vi "UHR-Fleezers Control (host) - 12.0_test_fpga_connection.vi"() -> ()   [LabVIEW 2014] (continued)
            n1532 = VISA Write(VISA resource name=w2158, write buffer=w2147) -> (VISA resource name out=w2146:refnum<visa-resource-name>)  [unwired: 1 in, 2 out]
            n1533 = Concatenate Strings("cvolume" ("string"), "\r") -> (w2145:string)
            n1534 = VISA Write(VISA resource name=w2146, write buffer=w2145) -> (VISA resource name out=w2156:refnum<visa-resource-name>)  [unwired: 1 in, 2 out]
            n1535 = Concatenate Strings("irun" ("string"), "\r") -> (w2154:string)
            n1536 = VISA Write(VISA resource name=w2156, write buffer=w2154) -> ()  [unwired: 1 in, 3 out]
          }
          frame #1 {
            "Flushing P3" <- TRUE ("Flushing P3")
          }
        }
      }
      event "Flush Pump 1": Value Change {
        n1537 = event-data() -> ()  [unwired: 7 out]
        n1538 = flat-sequence {
          tunnel: [w2176] -> w2166
          tunnel: w2165 -> [w2169]
          tunnel: w2166 -> [_]
          frame #0 {
            # "set paramaters (rate, volume) for flush, clear volume"
            n1539 = local write "Inject Pump 1"(TRUE ("Inject Pump 1")) -> ()
            n1540 = Number To Decimal String(number="Flush rate (uL/m) P1") -> (decimal integer string=w2192:string)  [unwired: 1 in]
            n1541 = Concatenate Strings("irate  " ("string"), w2192, " u/m" ("string"), "\r") -> (w2194:string)
            n1542 = VISA Write(VISA resource name=w2169, write buffer=w2194) -> (VISA resource name out=w2190:refnum<visa-resource-name>)  [unwired: 1 in, 2 out]
            n1543 = Reciprocal(x="Flush rate (uL/m) P1") -> (1/x=w2173:dbl)
            n1544 = Number To Decimal String(number="Volume (uL) P1") -> (decimal integer string=w2181:string)  [unwired: 1 in]
            n1545 = Multiply(x="Volume (uL) P1", y=w2173) -> (x*y=w2172:dbl)
            n1546 = Concatenate Strings("tvolume  " ("string"), w2181, " u" ("string"), "\r") -> (w2179:string)
            n1547 = Multiply(x=w2172, y=60.0) -> (x*y=→"HP1 Flush Time (s)":dbl)
            n1548 = VISA Write(VISA resource name=w2190, write buffer=w2179) -> (VISA resource name out=w2178:refnum<visa-resource-name>)  [unwired: 1 in, 2 out]
            n1549 = Concatenate Strings("cvolume" ("string"), "\r") -> (w2177:string)
            n1550 = VISA Write(VISA resource name=w2178, write buffer=w2177) -> (VISA resource name out=w2188:refnum<visa-resource-name>)  [unwired: 1 in, 2 out]
            n1551 = Concatenate Strings("irun" ("string"), "\r") -> (w2186:string)
            n1552 = VISA Write(VISA resource name=w2188, write buffer=w2186) -> (VISA resource name out=w2176:refnum<visa-resource-name>)  [unwired: 1 in, 2 out]
          }
          frame #1 {
            "Flushing P1" <- TRUE ("Flushing P3")
          }
        }
      }
      event "Clear Volume": Value Change {
        n1553 = event-data() -> ()  [unwired: 7 out]
        n1554 = Number To Decimal String(number="Normal volume (mL)") -> (decimal integer string=w2201:string)  [unwired: 1 in]
        n1555 = Concatenate Strings("tvolume " ("string"), w2201, " u" ("string"), "\r") -> (w2198:string)
        n1556 = VISA Write(VISA resource name=w2204, write buffer=w2198) -> (VISA resource name out=w2197:refnum<visa-resource-name>)  [unwired: 1 in, 2 out]
        n1557 = local write "Clear Volume"(FALSE ("Clear Volume")) -> ()
        n1558 = Concatenate Strings("cvolume" ("string"), "\r") -> (w2206:string)
        n1559 = VISA Write(VISA resource name=w2197, write buffer=w2206) -> ()  [unwired: 1 in, 3 out]
      }
      event "Clear Volume P3": Value Change {
        n1560 = event-data() -> ()  [unwired: 7 out]
        n1561 = Concatenate Strings("cvolume" ("string"), "\r") -> (w2212:string)
        n1562 = VISA Write(VISA resource name=w2211, write buffer=w2212) -> ()  [unwired: 1 in, 3 out]
        n1563 = local write "Clear Volume P3"(FALSE ("Clear Volume P3")) -> ()
      }
      event "Clear Volume P1": Value Change {
        n1564 = event-data() -> ()  [unwired: 7 out]
        n1565 = Concatenate Strings("cvolume" ("string"), "\r") -> (w2217:string)
        n1566 = local write "Clear Volume P1"(FALSE ("Clear Volume P1")) -> ()
        n1567 = VISA Write(VISA resource name=w2216, write buffer=w2217) -> ()  [unwired: 1 in, 3 out]
      }
      event "Display On P3": Value Change {
        n1568 = event-data() -> ()  [unwired: 7 out]
        n1569 = Select(t="dim 100", s="Display On P3", f="dim 0") -> (s? t:f=w2223:string)
        n1570 = Concatenate Strings(w2223, "\r") -> (w2225:string)
        n1571 = VISA Write(VISA resource name=w2220, write buffer=w2225) -> ()  [unwired: 1 in, 3 out]
      }
      event "Display On P1": Value Change {
        n1572 = event-data() -> ()  [unwired: 7 out]
        n1573 = Select(t="dim 100", s="Display On P1", f="dim 0") -> (s? t:f=w2230:string)
        n1574 = Concatenate Strings(w2230, "\r") -> (w2232:string)
        n1575 = VISA Write(VISA resource name=w2227, write buffer=w2232) -> ()  [unwired: 1 in, 3 out]
      }
      event "Retract Pump 3": Value Change {
        n1576 = event-data() -> ()  [unwired: 7 out]
        n1577 = local write "Retract Pump 3"(FALSE ("Retract Pump 3")) -> ()
        n1578 = case shown="True" "Retract Pump 3" {
          tunnel: w2234 -> [_ w2237]
          frame False {
          }
          frame True {
            n1579 = Number To Decimal String(number="Retract Rate (mL/m)") -> (decimal integer string=w2255:string)  [unwired: 1 in]
            n1580 = Concatenate Strings("wrate  " ("string"), w2255, " u/m" ("string"), "\r") -> (w2257:string)
            n1581 = VISA Write(VISA resource name=w2237, write buffer=w2257) -> (VISA resource name out=w2248:refnum<visa-resource-name>)  [unwired: 1 in, 2 out]
            n1582 = Number To Decimal String(number="Retract Vol 3 (uL)") -> (decimal integer string=w2250:string)  [unwired: 1 in]
            n1583 = Concatenate Strings("tvolume  " ("string"), w2250, " u" ("string"), "\r") -> (w2247:string)
            n1584 = VISA Write(VISA resource name=w2248, write buffer=w2247) -> (VISA resource name out=w2243:refnum<visa-resource-name>)  [unwired: 1 in, 2 out]
            n1585 = Concatenate Strings("cvolume" ("string"), "\r") -> (w2244:string)
            n1586 = VISA Write(VISA resource name=w2243, write buffer=w2244) -> (VISA resource name out=w2238:refnum<visa-resource-name>)  [unwired: 1 in, 2 out]
            n1587 = Concatenate Strings("wrun" ("string"), "\r") -> (w2239:string)
            n1588 = VISA Write(VISA resource name=w2238, write buffer=w2239) -> ()  [unwired: 1 in, 3 out]
          }
        }
      }
      event "Retract Pump 1": Value Change {
        n1589 = event-data() -> ()  [unwired: 7 out]
        n1590 = local write "Retract Pump 1"(FALSE ("Retract Pump 1")) -> ()
        n1591 = case shown="True" "Retract Pump 1" {
          tunnel: w2259 -> [_ w2264]
          frame False {
          }
          frame True {
            n1592 = local read "Retract Rate (mL/m)"() -> (w2262:dbl)
            n1593 = Number To Decimal String(number=w2262) -> (decimal integer string=w2280:string)  [unwired: 1 in]
            n1594 = Concatenate Strings("wrate  " ("string"), w2280, " u/m" ("string"), "\r") -> (w2282:string)
            n1595 = VISA Write(VISA resource name=w2264, write buffer=w2282) -> (VISA resource name out=w2274:refnum<visa-resource-name>)  [unwired: 1 in, 2 out]
            n1596 = Number To Decimal String(number="Retract Vol 1 (uL)") -> (decimal integer string=w2276:string)  [unwired: 1 in]
            n1597 = Concatenate Strings("tvolume  " ("string"), w2276, " u" ("string"), "\r") -> (w2273:string)
            n1598 = VISA Write(VISA resource name=w2274, write buffer=w2273) -> (VISA resource name out=w2270:refnum<visa-resource-name>)  [unwired: 1 in, 2 out]
            n1599 = Concatenate Strings("cvolume" ("string"), "\r") -> (w2271:string)
            n1600 = VISA Write(VISA resource name=w2270, write buffer=w2271) -> (VISA resource name out=w2265:refnum<visa-resource-name>)  [unwired: 1 in, 2 out]
            n1601 = Concatenate Strings("wrun" ("string"), "\r") -> (w2266:string)
            n1602 = VISA Write(VISA resource name=w2265, write buffer=w2266) -> ()  [unwired: 1 in, 3 out]
          }
        }
      }
      event "Flip Green Filter": Value Change {
        n1603 = event-data() -> ()  [unwired: 7 out]
        n1604 = Not(x="Flip Green Filter") -> (.not. x?=w2284:bool)
        n1605 = local write "Flip Green Filter"(w2284) -> ()
        n1606 = flat-sequence {
          tunnel: w2292 -> [w2297]
          tunnel: w2291 -> [w2296]
          tunnel: [w2294] -> w2289
          tunnel: [w2293] -> w2288
          tunnel: [w2299] -> w2287
          tunnel: w2289 -> [w2299]
          tunnel: [w2298] -> w2286
          tunnel: w2288 -> [w2298]
          tunnel: w2287 -> [w2303]
          tunnel: w2286 -> [w2302]
          tunnel: [w2301] -> w2290
          frame #0 {
            n1607 = xnode "Read/Write Control"("FPGA VI Reference In"=w2297, "error in"=w2296, "Green Filter Flipper"=TRUE) -> ("FPGA VI Reference Out"=w2294:T22, "error out"=w2293:errorcluster)
          }
          frame #1 {
            n1608 = Wait (ms)(milliseconds to wait=u32 100) -> ()  [unwired: 1 out]
          }
          frame #2 {
            n1609 = xnode "Read/Write Control"("FPGA VI Reference In"=w2303, "error in"=w2302, "Green Filter Flipper"=FALSE) -> ("error out"=w2301:errorcluster)  [unwired: 1 out]
          }
        }
      }
      event "Pump 1 contents", "Pump 3 contents": Value Change {
        n1610 = event-data() -> ()  [unwired: 7 out]
        n1611 = local read "Pump 1 contents"() -> (→"Pump 1 cont disp":string)
        n1612 = local read "Pump 3 contents"() -> (→"Pump 3 cont disp":string)
      }
      event "Reset Trap Pos. FB": Value Change {
        n1613 = event-data() -> ()  [unwired: 7 out]
        n1614 = xnode "Read/Write Control"("FPGA VI Reference In"=w2309, "error in"=w2308, "Trap Pos. FB Reset"="Reset Trap Pos. FB") -> ()  [unwired: 2 out]
      }
      event "Rem fb disp offset": Value Change {
        n1615 = event-data() -> ()  [unwired: 7 out]
        n1616 = local write "Rem fb disp offset"(FALSE ("Rem fb disp offset")) -> ()
        n1617 = local read "Mean T1 Position (nm)"() -> (w2311:dbl)
        n1618 = local read "FB Trap Pos Offset"() -> (w2312:dbl)
        n1619 = Subtract(x=w2312, y=w2311) -> (x-y=w2310:dbl)
        n1620 = local write "FB Trap Pos Offset"(w2310) -> ()
      }
      event "Threshold (nm)": Value Change {
        n1621 = event-data() -> ()  [unwired: 7 out]
        n1622 = flat-sequence {
          tunnel: w2316 -> [w2324]
          tunnel: w2315 -> [w2323]
          tunnel: [w2317] -> w2314
          tunnel: w2314 -> [w2330]
          frame #0 {
            n1623 = xnode "Read/Write Control"("FPGA VI Reference In"=w2324, "error in"=w2323) -> ("FPGA VI Reference Out"=w2320:T22, "error out"=w2319:errorcluster, "FPGA TTrig Thresh"=w2321:i64)
            n1624 = local read "Threshold stored (nm)"() -> (w2329:dbl)
            n1625 = local read "Threshold (nm)"() -> (w2317:dbl)
            n1626 = local read "AOM X Cal (nm/MHz)"() -> (w2327:dbl)
            n1627 = Subtract(x=w2317, y=w2329) -> (x-y=w2328:dbl)
            n1628 = Divide(x=w2328, y=w2327) -> (x/y=w2325:dbl)
            n1629 = call "IR AOM freq to word.vi"("Frequency In (MHz)"=w2325) -> ("Frequency Word Out (double)"=w2326:dbl)
            n1630 = To Quad Integer(1:w2326) -> (0:w2322:i64)
            n1631 = Add(x=w2321, y=w2322) -> (x+y=w2318:i64)
            n1632 = xnode "Read/Write Control"("FPGA VI Reference In"=w2320, "error in"=w2319, "FPGA TTrig Thresh"=w2318) -> ()  [unwired: 2 out]
          }
          frame #1 {
            "Threshold stored (nm)" <- w2330
          }
        }
      }
      event "FB Trig Integrate": Value Change {
        n1633 = event-data() -> ()  [unwired: 7 out]
        n1634 = local read "FB Trig Integrate"() -> (w2332:u32)
        n1635 = xnode "Read/Write Control"("FPGA VI Reference In"=w2334, "error in"=w2333, "FB Trig Integrate"=w2332) -> ("error out"=w2331:errorcluster)  [unwired: 1 out]
      }
      event "11": Value Change {
        n1636 = event-data() -> ()  [unwired: 7 out]
        n1637 = local read "11"() -> (w2335:bool)
        n1638 = case shown="True" w2335 {
          frame False {
          }
          frame True {
            n1639 = local read "Messages"() -> (w2337:string)
            n1640 = call "Update messages.vi"("Message to add"="You kicked it up to 11!", "Old message string"=w2337) -> ("New message string"=w2338:string)
            n1641 = call <vilib>:"Beep.vi"() -> ()  [unwired: 12 in]
            n1642 = local write "Messages"(w2338) -> ()
          }
        }
      }
      event "Trap Pos. FB ON": Value Change {
        n1643 = event-data() -> ()  [unwired: 7 out]
        n1644 = xnode "Read/Write Control"("FPGA VI Reference In"=w2341, "error in"=w2340, "Force feedback"="Trap Pos. FB ON") -> ()  [unwired: 2 out]
      }
      event "Remove Action Offset": Value Change {
        n1645 = event-data() -> ()  [unwired: 7 out]
        n1646 = local write "Remove Action Offset"(FALSE ("Remove Action Offset")) -> ()
        n1647 = local read "Trap Pos. FB Mult Factor"() -> (w2346:i64)
        n1648 = local read "Trap Pos FB Action"() -> (w2344:i64)
        n1649 = local read "Trap Pos. FB Offset Factor"() -> (w2342:i64)
        n1650 = Multiply(x=w2346, y=w2344) -> (x*y=w2345:i64)
        n1651 = Add(x=w2345, y=w2342) -> (x+y=w2343:i64)
        n1652 = local write "Trap Pos. FB Offset Factor"(w2343) -> ()
        n1653 = xnode "Read/Write Control"("FPGA VI Reference In"=w2349, "error in"=w2348, "Trap Pos. FB Offset Factor"=w2343) -> ()  [unwired: 2 out]
      }
      event "Remove Offset to factor": Value Change {
        n1654 = event-data() -> ()  [unwired: 7 out]
        n1655 = local write "Remove Offset to factor"(FALSE ("Remove Action Offset")) -> ()
        n1656 = local read "Trap Pos. FB Mult Factor"() -> (w2361:i64)
        n1657 = local read "Trap Pos FB Action"() -> (w2359:i64)
        n1658 = local read "Trap Pos. FB Offset Factor"() -> (w2358:i64)
        n1659 = Multiply(x=w2361, y=w2359) -> (x*y=w2360:i64)
        n1660 = local read "Trap Pos. FB Mult Factor"() -> (w2357:i64)
        n1661 = Add(x=w2360, y=w2358) -> (x+y=w2352:i64)
        n1662 = Multiply(x=32768, y="factor") -> (x*y=w2355:dbl)
        n1663 = Multiply(x=w2355, y=w2357) -> (x*y=w2356:dbl)
        n1664 = Subtract(x=w2352, y=w2356) -> (x-y=w2350:dbl)
        n1665 = To Quad Integer(1:w2350) -> (0:w2351:i64)
        n1666 = xnode "Read/Write Control"("FPGA VI Reference In"=w2364, "error in"=w2363, "Trap Pos. FB Offset Factor"=w2351) -> ()  [unwired: 2 out]
        n1667 = local write "Trap Pos. FB Offset Factor"(w2351) -> ()
      }
      event "Trap Pos. FB Range", "Trap Pos. FB Gains", "Trap Pos. FB Mult Factor", "Trap Pos. FB Offset Factor", "Trap Pos FB Negate Action", "Trap Pos FB Monitor\nT1 or T2", "Differential FB?", "Negate Diff?": Value Change {
        n1668 = event-data() -> ()  [unwired: 7 out]
        n1669 = local read "Negate Diff?"() -> (w2365:bool)
        n1670 = xnode "Read/Write Control"("FPGA VI Reference In"=w2375, "error in"=w2374, "Trap Pos. FB Range"="Trap Pos. FB Range", "Trap Pos. FB Gains"="Trap Pos. FB Gains", "Trap Pos. FB Mult Factor"="Trap Pos. FB Mult Factor", "Trap Pos. FB Offset Factor"="Trap Pos. FB Offset Factor", "Trap Pos FB Negate Action"="Trap Pos FB Negate Action", "Trap Pos FB Monitor T1 or T2"="Trap Pos FB Monitor\nT1 or T2", "AI1 X Scale"="Trap Pos. AI1 X Pre-scale", "Negate Diff?"=w2365, "Diff FB Measurement?"="Differential FB?") -> ()  [unwired: 2 out]
      }
      event "Trap Pos FB SP", "Trap Pos FB SP 2", "Use SP 2": Value Change {
        n1671 = event-data() -> ()  [unwired: 7 out]
        n1672 = Select(t="Trap Pos FB SP 2", s="Use SP 2", f="Trap Pos FB SP") -> (s? t:f=w2376:fxp<+/-,16,1>)
        n1673 = xnode "Read/Write Control"("FPGA VI Reference In"=w2381, "error in"=w2380, "Trap Pos. FB SP"=w2376) -> ()  [unwired: 2 out]
      }
      event "Offset SP2 from SP1": Value Change {
        n1674 = event-data() -> ()  [unwired: 7 out]
        n1675 = local read "Trap Pos FB SP"() -> (w2384:fxp<+/-,16,1>)
        n1676 = Add(x=w2384, y="SP2 Offset") -> (x+y=w2382:fxp<+/-,16,1>)
        n1677 = property on="Trap Pos FB SP 2" class="DigNum (strict)"("Val(Sgnl)"=w2382) -> ()  [unwired: 2 in, 2 out]
        n1678 = local write "Offset SP2 from SP1"(FALSE ("Offset SP2 from SP1")) -> ()
      }
      event "Set Reading to\nSetpoint": Value Change {
        # "This is the actual PID input signal"
        n1679 = event-data() -> ()  [unwired: 7 out]
        n1680 = local write "Set Reading to\nSetpoint"(FALSE ("Set SP to Reading")) -> ()
        n1681 = xnode "Read/Write Control"("FPGA VI Reference In"=w2390, "error in"=w2389) -> ("FPGA VI Reference Out"=w2388:T22, "error out"=w2387:errorcluster, "Trap Pos FB Int-Norm Signal"=w2386:fxp<+/-,16,1>)
        n1682 = local read "Differential FB?"() -> (w2391:bool)
        n1683 = case shown="False" w2391 {
          tunnel: [w2396 w2403] -> w2393
          tunnel: w2386 -> [w2394 w2403]
          frame False {
            n1684 = local read "Trap Pos FB Monitor\nT1 or T2"() -> (w2399:bool)
            n1685 = local read "Trap X AI1 (DMA)"() -> (w2402:T13)
            n1686 = Unbundle By Name(w2402) -> ("Set 1"=w2401:fxp<+/-,16,1>, "Set 2"=w2400:fxp<+/-,16,1>)
            n1687 = Select(t=w2401, s=w2399, f=w2400) -> (s? t:f=w2398:fxp<+/-,16,1>)
            n1688 = Not(x="Set SP Using...") -> (.not. x?=w2395:bool)
            n1689 = Select(t=w2394, s=w2395, f=w2398) -> (s? t:f=w2396:fxp<+/-,16,1>)
          }
          frame True {
          }
        }
        n1690 = xnode "Read/Write Control"("FPGA VI Reference In"=w2388, "error in"=w2387, "Trap Pos. FB SP"=w2393) -> ()  [unwired: 2 out]
        n1691 = local write "Trap Pos FB SP"(w2393) -> ()
      }
      event "Trap Pos. FB Out Scale 2^n": Value Change {
        n1692 = event-data() -> ()  [unwired: 7 out]
        n1693 = Scale By Power Of 2(n="Trap Pos. FB Out Scale 2^n", x=ext 1.0) -> (x*2^n=w2404:ext)
        n1694 = property on="Trap Pos. FB Mult Factor" class="DigNum (strict)"("Val(Sgnl)"=w2404) -> ()  [unwired: 2 in, 2 out]
      }
      event "Trap Pos FB Int Count": Value Change {
        n1695 = event-data() -> ()  [unwired: 7 out]
        n1696 = xnode "Read/Write Control"("FPGA VI Reference In"=w2409, "error in"=w2408, "Trap Pos FB Int Count"="Trap Pos FB Int Count") -> ()  [unwired: 2 out]
      }
      event "Trap pos": Value Change {
        n1697 = event-data() -> ()  [unwired: 7 out]
        n1698 = case shown="True" "Trap pos" {
          frame False {
            n1699 = property on="Trap Delta Graph" class="WFGraph (strict)"("Visible"=TRUE) -> ()  [unwired: 2 in, 2 out]
            n1700 = property on="Saved trap pos" class="WFGraph (strict)"("Visible"=FALSE) -> ()  [unwired: 2 in, 2 out]
          }
          frame True {
            n1701 = property on="Saved trap pos" class="WFGraph (strict)"("Visible"=TRUE) -> ()  [unwired: 2 in, 2 out]
            n1702 = property on="Trap Delta Graph" class="WFGraph (strict)"("Visible"=FALSE) -> ()  [unwired: 2 in, 2 out]
          }
        }
      }
      event "Save user params": Value Change {
        n1703 = event-data() -> ()  [unwired: 7 out]
        n1704 = local write "Save user params"(FALSE ("Save user\nparams")) -> ()
        n1705 = call "save control values.vi"("User"="User") -> ()  [unwired: 8 in, 1 out]
        n1706 = local read "Messages"() -> (w2421:string)
        n1707 = Concatenate Strings("User: ", "User", "\r", "Parameters saved.") -> (w2416:string)
        n1708 = call "Update messages.vi"("Message to add"=w2416, "Old message string"=w2421) -> ("New message string"=w2415:string)
        n1709 = local write "Messages"(w2415) -> ()
      }
      event "Load user params": Value Change {
        n1710 = event-data() -> ()  [unwired: 7 out]
        n1711 = local write "Load user params"(FALSE ("Read user\nparams")) -> ()
        n1712 = flat-sequence {
          tunnel: [w2453] -> w2441
          tunnel: [w2452] -> w2439
          tunnel: [w2451] -> w2437
          tunnel: [w2450] -> w2435
          tunnel: [w2449] -> w2433
          tunnel: [w2448] -> w2431
          tunnel: [w2447] -> w2429
          tunnel: [w2446] -> w2427
          tunnel: [w2445] -> w2425
          tunnel: [w2444] -> w2423
          tunnel: [w2463] -> w2442
          tunnel: w2441 -> [w2463]
          tunnel: [w2462] -> w2440
          tunnel: w2439 -> [w2462]
          tunnel: [w2461] -> w2438
          tunnel: w2437 -> [w2461]
          tunnel: [w2460] -> w2436
          tunnel: w2435 -> [w2460]
          tunnel: [w2459] -> w2434
          tunnel: w2433 -> [w2459]
          tunnel: [w2458] -> w2432
          tunnel: w2431 -> [w2458]
          tunnel: [w2457] -> w2430
          tunnel: w2429 -> [w2457]
          tunnel: [w2456] -> w2428
          tunnel: w2427 -> [w2456]
          tunnel: [w2455] -> w2426
          tunnel: w2425 -> [w2455]
          tunnel: [w2454] -> w2424
          tunnel: w2423 -> [w2454]
          tunnel: w2442 -> [w2480]
          tunnel: w2440 -> [w2479]
          tunnel: w2438 -> [w2478]
          tunnel: w2436 -> [w2477]
          tunnel: w2434 -> [w2476]
          tunnel: w2432 -> [w2475]
          tunnel: w2430 -> [w2474]
          tunnel: w2428 -> [w2473]
          tunnel: w2426 -> [w2472]
          tunnel: w2424 -> [w2471]
          frame #0 {
            # "Make exceptions.\nThese will not be\nloaded."
            n1713 = local read "Sample Channel\nFlow"() -> (w2448:bool)
            n1714 = local read "Green ON/Interlacing"() -> (w2449:bool)
            n1715 = local read "Trap 1 (ON/OFF)"() -> (w2453:bool)
            n1716 = local read "Trap 2 (ON/OFF)"() -> (w2452:bool)
            n1717 = local read "Trap Pos. FB ON"() -> (w2444:bool)
            n1718 = local read "Inject Pump 1"() -> (w2447:bool)
            n1719 = local read "Inject Pump 3"() -> (w2446:bool)
            n1720 = local read "Trap D (MHz)"() -> (w2445:dbl)
            n1721 = local read "Index"() -> (w2450:dbl)
            n1722 = local read "Fish"() -> (w2451:bool)
          }
          frame #1 {
            n1723 = local read "User"() -> (w2464:string)
            n1724 = call "retrieve control values.vi"("User"=w2464) -> ()  [unwired: 10 in, 1 out]
            n1725 = local read "Messages"() -> (w2470:string)
            n1726 = Concatenate Strings("User: ", w2464, "\r", "Parameters loaded.") -> (w2465:string)
            n1727 = call "Update messages.vi"("Message to add"=w2465, "Old message string"=w2470) -> ("New message string"=w2469:string)
            n1728 = local write "Messages"(w2469) -> ()
          }
          frame #2 {
            n1729 = local write "Sample Channel\nFlow"(w2475) -> ()
            n1730 = local write "Green ON/Interlacing"(w2476) -> ()
            n1731 = local write "Trap 1 (ON/OFF)"(w2480) -> ()
            n1732 = local write "Trap 2 (ON/OFF)"(w2479) -> ()
            n1733 = local write "Inject Pump 1"(w2474) -> ()
            n1734 = local write "Trap Pos. FB ON"(w2471) -> ()
            n1735 = local write "Inject Pump 3"(w2473) -> ()
            n1736 = local write "Trap D (MHz)"(w2472) -> ()
            n1737 = local write "Index"(w2477) -> ()
            n1738 = local write "Fish"(w2478) -> ()
          }
        }
      }
      event "Abort wiggle": Value Change {
        n1739 = event-data() -> ()  [unwired: 7 out]
        n1740 = flat-sequence {
          tunnel: w2484 -> [w2488]
          tunnel: w2483 -> [w2487]
          tunnel: [w2486] -> w2481
          tunnel: [w2490] -> w2482
          tunnel: w2481 -> [w2490]
          frame #0 {
            n1741 = xnode "Read/Write Control"("FPGA VI Reference In"=w2488, "error in"=w2487, "Abort wiggle 1"="Abort wiggle", "Abort wiggle 2"="Abort wiggle") -> ("error out"=w2486:errorcluster)  [unwired: 1 out]
          }
          frame #1 {
            n1742 = local write "Abort wiggle"(FALSE ("Abort wiggle")) -> ()
          }
        }
      }
    }
    "error out 2" <- w1261
    n1743 = node-c288() -> ()  [unwired: 2 out]
  }
  n1744 = node-c288() -> (w126:T26)  [unwired: 4 in]
  n1745 = local write "Target size"(cluster{"Width":dbl, "Height":dbl} {"Width"=40.0, "Height"=40.0} ("Target size")) -> ()
  n1746 = timed-loop "Run Scripts, including: stage motion" {
    tunnel: w130 -> [w2498]
    tunnel: w5 -> [w2499]
    tunnel: [w2499] -> w129
    tunnel: [w2498] -> w128
    timing: w126 -> [_]
    timing-out: [_] -> w125
    tunnel: w111 -> [w2497]
    tunnel: w112 -> [w2496]
    tunnel: w55 -> [w2493]
    tunnel: w54 -> [w2492]
    tunnel: w53 -> [w2494]
    tunnel: w52 -> [w2495]
    stop <- w2491 stop-if-true
    n1747 = node-c288() -> ()  [unwired: 1 in, 1 out]
    n1748 = event shown="[12] \"Got ADig bead\": Value Change" {
      selector: _ -> [_ _ _ _ _ _ _ _ _ _ _ _ _ _ _ _ _ _ _ _ _]
      dyn-events: _ -> [_ _ _ _ _ _ _ _ _ _ _ _ _ _ _ _ _ _ _ _ _]
      timeout: _ -> [_ _ _ _ _ _ _ _ _ _ _ _ _ _ _ _ _ _ _ _ _]
      tunnel: ["Set Position" "Move to Position" _ _ "Read Harvard" _ _ _ _ _ _ _ "Got ADig bead" "Force FB Script" "Rupture Script" _ "Got DNA bead" "Take Stepping Data" _ "Take Detection Laser\nImage" _] -> _
      tunnel: [_ _ _ _ _ _ _ _ _ _ _ _ _ _ _ _ _ _ _ _ w3172] -> w2491
      tunnel: w2498 -> [w2517 w2525 w2538 w2568 _ w2616 w2656 w2739 w2770 w2904 w2930 w2965 _ w2983 _ _ _ _ _ _ _]
      tunnel: w2499 -> [w2518 w2526 w2539 w2569 _ w2617 w2657 w2740 w2771 w2905 w2931 w2966 _ w2984 _ _ _ _ _ _ _]
      tunnel: w2497 -> [_ _ _ _ w2601 _ _ _ _ _ _ _ _ _ _ _ _ _ _ _ _]
      tunnel: w2496 -> [_ _ _ _ w2600 _ _ _ _ _ _ _ _ _ _ _ _ _ _ _ _]
      tunnel: w2495 -> [_ _ _ _ _ _ _ _ _ _ _ _ _ _ _ _ _ _ _ _ _]
      tunnel: w2494 -> [_ _ _ _ _ _ _ _ _ _ _ _ _ _ _ _ _ _ _ _ _]
      tunnel: w2493 -> [_ _ _ _ _ _ _ _ _ _ _ _ _ _ _ _ _ _ _ _ _]
      tunnel: w2492 -> [_ _ _ _ _ _ _ _ _ _ _ _ _ _ _ _ _ _ _ _ _]
      event "Set Position", "Set Position 2", "Set Position 3", "Set Position 4", "Set Position 5", "Set Position 1": Value Change {
        n1749 = event-data() -> ()  [unwired: 1 in, 5 out]
        n1750 = Build Array("Set Position 1", "Set Position 2", "Set Position 3", "Set Position 4", "Set Position 5") -> (w2516:bool[])
        n1751 = Boolean Array To Number(Boolean array=w2516) -> (number=w2515:u32)
        n1752 = Logarithm Base 2(1:w2515) -> (0:w2507:dbl)
        n1753 = call "Read Stage Position.vi"("error in"=w2517, "VISA resource name in"=w2518) -> ("Current Position"=w2522:cluster{dbl, dbl, dbl}, "error out"=w2521:errorcluster)  [unwired: 2 out]
        n1754 = Decrement(x="Position") -> (x-1=w2505:dbl)
        n1755 = Greater Or Equal?(x=w2507, y=0.0) -> (x >= y?=w2508:bool)
        n1756 = Cluster To Array(cluster=w2522) -> (array=w2519:dbl[])
        n1757 = local write "Stage Control Serial Error"(w2521) -> ()
        n1758 = Select(t=w2507, s=w2508, f=w2505) -> (s? t:f=w2504:dbl)
        n1759 = Increment(x=w2504) -> (x+1=w2503:dbl)
        n1760 = Build Array (concatenate)(w2503, w2519) -> (w2502:dbl[])
        n1761 = Replace Array Subset(array="Saved Stage Positions", new element=w2502, index (row)=w2504) -> (w2520:dbl[][])  [unwired: 1 in]
        n1762 = local write "Saved Stage Positions"(w2520) -> ()
      }
      event "Move to Position": Value Change {
        n1763 = event-data() -> ()  [unwired: 1 in, 5 out]
        n1764 = flat-sequence {
          tunnel: w2526 -> [w2530]
          tunnel: w2525 -> [w2529]
          frame #0 {
            n1765 = local read "Saved Stage Positions"() -> (w2532:dbl[][])
            n1766 = local read "Position"() -> (w2531:dbl)
            n1767 = local write "Stage Moving"(TRUE ("Stage Moving")) -> ()
            n1768 = call "move to saved stage position.vi"("error in"=w2529, "Stage VISA resource name in"=w2530, "Position"=w2531, "Saved Stage Positions"=w2532) -> ("error out"=w2528:errorcluster)  [unwired: 1 out]
            n1769 = local write "Stage Control Serial Error"(w2528) -> ()
          }
          frame #1 {
            n1770 = call <vilib>:"Beep.vi"() -> ()  [unwired: 3 in, 9 out]
            n1771 = local write "Stage Moving"(FALSE ("Stage Moving")) -> ()
          }
        }
      }
      event "Move Cap. 1 (DNA Bottom)": Value Change {
        n1772 = event-data() -> ()  [unwired: 1 in, 5 out]
        n1773 = local write "Move Cap. 1 (DNA Bottom)"(FALSE ("Move Cap. 1 (DNA Right)")) -> ()
        n1774 = flat-sequence {
          tunnel: w2538 -> [w2541]
          tunnel: w2539 -> [w2542]
          tunnel: [w2542] -> w2536
          tunnel: [w2541] -> w2535
          tunnel: w2536 -> [w2544]
          tunnel: w2535 -> [w2543]
          frame #0 {
            n1775 = property on="Sample Channel\nFlow" class="Bool (strict)"("Val(Sgnl)"="Cap 1 Samp Flow ON") -> ()  [unwired: 2 in, 2 out]
          }
          frame #1 {
            n1776 = local read "Saved Stage Positions"() -> (w2554:dbl[][])
            n1777 = local write "Stage Moving"(TRUE ("Stage Moving")) -> ()
            n1778 = Array Subset(array=w2554, index (row)=0 ("index"), length (row)=1 ("length"), index (col)=1 ("index"), length (col)=3 ("length")) -> (w2551:dbl[][])
            n1779 = Reshape Array(w2551, 3 ("dimension size")) -> (w2549:dbl[])
            n1780 = Array To Cluster(array=w2549) -> (cluster=w2548:cluster{"[0]":dbl, "[1]":dbl, "[2]":dbl})
            n1781 = call "Set Stage Position.vi"("Position"=w2548, "error in"=w2543, "VISA resource name in"=w2544) -> ("error out"=w2547:errorcluster)  [unwired: 2 out]
            n1782 = local write "Stage Control Serial Error"(w2547) -> ()
          }
          frame #2 {
            n1783 = local write "Stage Moving"(FALSE ("Stage Moving")) -> ()
            n1784 = case shown="True" "Cap 1 Flow ON" {
              frame False {
              }
              frame True {
                n1785 = property on="Inject Pump 1" class="Bool (strict)"("Val(Sgnl)"=TRUE ("Value (Signaling)")) -> ()  [unwired: 2 in, 2 out]
              }
            }
            n1786 = call <vilib>:"Beep.vi"() -> ()  [unwired: 3 in, 9 out]
          }
          frame #3 {
            n1787 = property on="Sample Channel\nFlow" class="Bool (strict)"("Val(Sgnl)"=FALSE ("Value (Signaling)")) -> ()  [unwired: 2 in, 2 out]
            n1788 = local read "Cap. 2 BD T1?\n(ADig T1, DNA T2)"() -> (w2561:bool)
            n1789 = case shown="True" w2561 {
              tunnel: "Cap 1 T ON" -> [w2563 w2564]
              frame False {
                n1790 = property on="Trap 1 (ON/OFF)" class="Bool (strict)"("Val(Sgnl)"=w2563) -> ()  [unwired: 2 in, 2 out]
              }
              frame True {
                n1791 = property on="Trap 2 (ON/OFF)" class="Bool (strict)"("Val(Sgnl)"=w2564) -> ()  [unwired: 2 in, 2 out]
              }
            }
            n1792 = property on="Got DNA bead" class="Bool (strict)"("Key Focus"=TRUE) -> ()  [unwired: 2 in, 2 out]
          }
        }
      }
      event "Move Cap. 2 (ADig Top)": Value Change {
        n1793 = event-data() -> ()  [unwired: 1 in, 5 out]
        n1794 = local write "Move Cap. 2 (ADig Top)"(FALSE ("Move Cap. 2 (ADig Left)")) -> ()
        n1795 = flat-sequence {
          tunnel: w2568 -> [w2571]
          tunnel: w2569 -> [w2572]
          tunnel: [w2572] -> w2566
          tunnel: [w2571] -> w2565
          tunnel: w2566 -> [w2574]
          tunnel: w2565 -> [w2573]
          frame #0 {
            n1796 = property on="Sample Channel\nFlow" class="Bool (strict)"("Val(Sgnl)"="Cap 2 Samp Flow ON") -> ()  [unwired: 2 in, 2 out]
          }
          frame #1 {
            n1797 = local read "Saved Stage Positions"() -> (w2584:dbl[][])
            n1798 = local write "Stage Moving"(TRUE ("Stage Moving")) -> ()
            n1799 = Array Subset(array=w2584, index (row)=1 ("index"), length (row)=1 ("length"), index (col)=1 ("index"), length (col)=3 ("length")) -> (w2581:dbl[][])
            n1800 = disable-structure shown="Disabled" {
              frame Disabled {
                w2586 = FALSE ("Value (Signaling)")
                n1801 = property on="Trap 1 (ON/OFF)" class="Bool (strict)"("Val(Sgnl)"=w2586) -> ()  [unwired: 2 in, 2 out]
                n1802 = property on="Trap 1 (ON/OFF)" class="Bool (strict)"("Val(Sgnl)"=w2586) -> ()  [unwired: 2 in, 2 out]
              }
              frame Enabled {
              }
            }
            n1803 = Reshape Array(w2581, 3 ("dimension size")) -> (w2579:dbl[])
            n1804 = Array To Cluster(array=w2579) -> (cluster=w2578:cluster{"[0]":dbl, "[1]":dbl, "[2]":dbl})
            n1805 = call "Set Stage Position.vi"("Position"=w2578, "error in"=w2573, "VISA resource name in"=w2574) -> ("error out"=w2577:errorcluster)  [unwired: 2 out]
            n1806 = local write "Stage Control Serial Error"(w2577) -> ()
          }
          frame #2 {
            n1807 = local write "Stage Moving"(FALSE ("Stage Moving")) -> ()
            n1808 = call <vilib>:"Beep.vi"() -> ()  [unwired: 3 in, 9 out]
            n1809 = case shown="True" "Cap 2 Flow ON" {
              frame False {
              }
              frame True {
                n1810 = property on="Inject Pump 3" class="Bool (strict)"("Val(Sgnl)"=TRUE ("Value (Signaling)")) -> ()  [unwired: 2 in, 2 out]
              }
            }
          }
          frame #3 {
            n1811 = Wait (ms)(milliseconds to wait=u32 500) -> ()  [unwired: 1 out]
          }
          frame #4 {
            n1812 = local read "Cal @ (MHz)"() -> (w2592:dbl)
            n1813 = property on="Sample Channel\nFlow" class="Bool (strict)"("Val(Sgnl)"=FALSE ("Value (Signaling)")) -> ()  [unwired: 2 in, 2 out]
            n1814 = case shown="False" "Cap. 2 BD T1?\n(ADig T1, DNA T2)" {
              tunnel: "Cap 2 T ON" -> [w2597 w2598]
              frame False {
                n1815 = property on="Trap 2 (ON/OFF)" class="Bool (strict)"("Val(Sgnl)"=w2597) -> ()  [unwired: 2 in, 2 out]
              }
              frame True {
                n1816 = property on="Trap 1 (ON/OFF)" class="Bool (strict)"("Val(Sgnl)"=w2598) -> ()  [unwired: 2 in, 2 out]
              }
            }
            n1817 = property on="Got ADig bead" class="Bool (strict)"("Key Focus"=TRUE) -> ()  [unwired: 2 in, 2 out]
            n1818 = local write "Target"("Target\nON?") -> ()
            n1819 = property on="Trap D (MHz)" class="DigNum (strict)"("Val(Sgnl)"=w2592) -> ()  [unwired: 2 in, 2 out]
          }
        }
      }
      event "Read Harvard": Value Change {
        n1820 = event-data() -> ()  [unwired: 1 in, 5 out]
        n1821 = Concatenate Strings("write buffer", "\r") -> (w2603:string)
        n1822 = VISA Write(VISA resource name=w2601, write buffer=w2603, error in (no error)=w2600) -> (VISA resource name out=w2612:refnum<visa-resource-name>, error out=w2611:errorcluster)  [unwired: 1 out]
        n1823 = stacked-sequence {
          tunnel: [w2615] -> w2610
          tunnel: w2612 -> [w2615]
          tunnel: w2611 -> [w2614]
          tunnel: [w2614] -> w2605
          frame #0 {
            n1824 = Wait (ms)(milliseconds to wait=50) -> ()  [unwired: 1 out]
          }
        }
        n1825 = property class="Instr"(reference=w2610, error in=w2605) -> (reference out=w2609:refnum<visa-resource-name>, error out=w2607:errorcluster, "Serial Settings:Number of Bytes at Serial Port"=w2608:u32)
        "Serial Settings:Number of Bytes at Serial Port" <- w2608
        n1826 = VISA Read(VISA resource name=w2609, byte count=w2608, error in (no error)=w2607) -> (read buffer=w2606:string)  [unwired: 3 out]
        "read buffer" <- w2606
        n1827 = Fract/Exp String To Number(string=w2606) -> ()  [unwired: 5 out]
      }
      event "+z", "-z": Value Change {
        n1828 = event-data() -> ()  [unwired: 1 in, 5 out]
        n1829 = flat-sequence {
          tunnel: w2616 -> [w2638]
          tunnel: w2617 -> [w2618]
          frame #0 {
            n1830 = call "Read Stage Position.vi"("error in"=w2638, "VISA resource name in"=w2618) -> ("Current Position"=w2623:cluster{dbl, dbl, dbl}, "error out"=w2636:errorcluster, "VISA resource name out"=w2637:refnum<visa-resource-name>)  [unwired: 1 out]
            n1831 = local read "Saved Stage Positions"() -> (w2647:dbl[][])
            n1832 = Divide(x="z nudge increment (um)", y=1000.0) -> (x/y=w2635:dbl)
            n1833 = Boolean To (0,1)(Boolean="+z") -> (0, 1=w2627:i16)
            n1834 = Boolean To (0,1)(Boolean="-z") -> (0, 1=w2628:i16)
            n1835 = Array Subset(array=w2647, index (row)=1 ("index"), length (row)=1 ("length"), index (col)=1 ("index"), length (col)=3 ("length")) -> (w2644:dbl[][])
            n1836 = Multiply(x=w2627, y=w2635) -> (x*y=w2631:dbl)
            n1837 = Multiply(x=w2628, y=w2635) -> (x*y=w2629:dbl)
            n1838 = Unbundle(w2623) -> (w2621:dbl, w2620:dbl, w2624:dbl)
            n1839 = Negate(x=w2629) -> (-x=w2630:dbl)
            n1840 = Reshape Array(w2644, 3 ("dimension size")) -> (w2642:dbl[])
            n1841 = Add(x=w2631, y=w2630) -> (x+y=w2632:dbl)
            n1842 = Array To Cluster(array=w2642) -> ()  [unwired: 1 out]
            n1843 = Add(x=w2632, y=w2624) -> (x+y=w2622:dbl)
            n1844 = Bundle(cluster=w2623, w2621, w2620, w2622) -> (w2619:cluster{dbl, dbl, dbl})
            n1845 = call "Set Stage Position.vi"("Position"=w2619, "error in"=w2636, "VISA resource name in"=w2637) -> ("error out"=w2641:errorcluster)  [unwired: 2 out]
            n1846 = local write "Stage Moving"(TRUE ("Stage Moving")) -> ()
            n1847 = local write "Stage Control Serial Error"(w2641) -> ()
          }
          frame #1 {
            n1848 = local write "Stage Moving"(FALSE ("Stage Moving")) -> ()
            n1849 = call <vilib>:"Beep.vi"() -> ()  [unwired: 3 in, 9 out]
          }
        }
      }
      event "Cal/Data Acq. Spot": Value Change {
        n1850 = event-data() -> ()  [unwired: 1 in, 5 out]
        n1851 = flat-sequence {
          tunnel: w2656 -> [w2660]
          tunnel: w2657 -> [w2661]
          tunnel: [w2661] -> w2653
          tunnel: [w2660] -> w2652
          tunnel: w2653 -> [w2666]
          tunnel: w2652 -> [w2665]
          tunnel: ["Cal @ (MHz)"] -> w2650
          tunnel: [w2670] -> w2654
          tunnel: w2650 -> [w2670]
          tunnel: w2654 -> [w2681]
          tunnel: ["W/ Offset 1"] -> w2651
          tunnel: w2654 -> [w2702]
          tunnel: w2651 -> [w2700]
          frame #0 {
            n1852 = property on="Sample Channel\nFlow" class="Bool (strict)"("Val(Sgnl)"="Daq spot flow on") -> ()  [unwired: 2 in, 2 out]
            n1853 = Wait (ms)(milliseconds to wait=u32 250) -> ()  [unwired: 1 out]
          }
          frame #1 {
            n1854 = local read "Saved Stage Positions"() -> (w2663:dbl[][])
            n1855 = property on="Trap D (MHz)" class="DigNum (strict)"("Val(Sgnl)"="Cal @ (MHz)") -> ()  [unwired: 2 in, 2 out]
            n1856 = local write "Stage Moving"(TRUE ("Stage Moving")) -> ()
            n1857 = call "move to saved stage position.vi"("error in"=w2665, "Stage VISA resource name in"=w2666, "Position"="Cal Stage Position", "Saved Stage Positions"=w2663) -> ("error out"=w2664:errorcluster)  [unwired: 1 out]
            n1858 = local write "Stage Control Serial Error"(w2664) -> ()
          }
          frame #2 {
            n1859 = local write "Stage Moving"(FALSE ("Stage Moving")) -> ()
            n1860 = property on="Sample Channel\nFlow" class="Bool (strict)"("Val(Sgnl)"="Flow ON\nduring cal?") -> ()  [unwired: 2 in, 2 out]
            n1861 = call <vilib>:"Beep.vi"() -> ()  [unwired: 3 in, 9 out]
          }
          frame #3 {
            n1862 = local read "Wait Before Save (s)"() -> (w2673:u32)
            n1863 = Multiply(x=w2673, y=u32 1000 ("milliseconds to wait")) -> (x*y=w2674:u32)
            n1864 = Wait (ms)(milliseconds to wait=w2674) -> ()  [unwired: 1 out]
          }
          frame #4 {
            n1865 = property on="Save Calibration" class="Bool (strict)"("Val(Sgnl)"=TRUE ("Value (Signaling)")) -> ()  [unwired: 2 in, 2 out]
          }
          frame #5 {
            n1866 = Wait (ms)(milliseconds to wait=u32 2000) -> ()  [unwired: 1 out]
          }
          frame #6 {
            # "Check to see if \nsaving done"
            n1867 = while {
              stop <- w2677 stop-if-true
              n1868 = local read "Saving..."() -> (w2678:bool)
              n1869 = Wait (ms)(milliseconds to wait=u32 100) -> ()  [unwired: 1 out]
              n1870 = Not(x=w2678) -> (.not. x?=w2677:bool)
            }
          }
          frame #7 {
            n1871 = case shown="True" "W/ Offset 1" {
              tunnel: w2681 -> [_ w2682]
              frame False {
              }
              frame True {
                n1872 = stacked-sequence {
                  tunnel: w2682 -> [_ _ _ _ _ _ _ w2699]
                  frame #0 {
                    n1873 = property on="Trap D (MHz)" class="DigNum (strict)"("Val(Sgnl)"="Offset 1 Start (MHz)") -> ()  [unwired: 2 in, 2 out]
                    n1874 = Replace Array Subset(array=u32[] [0] ("Index Values"), new element="Offset 1 Set", index=0) -> (w2683:u32[])
                    n1875 = property on="Saved AOD Raster Scan Parameter Sets" class="Arr (strict)"("Index Values"=w2683) -> ()  [unwired: 2 in, 2 out]
                  }
                  frame #1 {
                    n1876 = Wait (ms)(milliseconds to wait=u32 200) -> ()  [unwired: 1 out]
                  }
                  frame #2 {
                    n1877 = property on="Load parameters" class="Bool (strict)"("Val(Sgnl)"=TRUE ("Value (Signaling)")) -> ()  [unwired: 2 in, 2 out]
                  }
                  frame #3 {
                    n1878 = Wait (ms)(milliseconds to wait=u32 200) -> ()  [unwired: 1 out]
                  }
                  frame #4 {
                    n1879 = property on="Trap Raster Scan" class="Bool (strict)"("Val(Sgnl)"=TRUE ("Value (Signaling)")) -> ()  [unwired: 2 in, 2 out]
                  }
                  frame #5 {
                    n1880 = Wait (ms)(milliseconds to wait=u32 2000) -> ()  [unwired: 1 out]
                  }
                  frame #6 {
                    n1881 = while {
                      stop <- w2696 stop-if-true
                      n1882 = local read "Raster Scanning..."() -> (w2698:bool)
                      n1883 = local read "Saving..."() -> (w2694:bool)
                      n1884 = Wait (ms)(milliseconds to wait=u32 100) -> ()  [unwired: 1 out]
                      n1885 = Not(x=w2694) -> (.not. x?=w2693:bool)
                      n1886 = Not(x=w2698) -> (.not. x?=w2695:bool)
                      n1887 = And(x=w2695, y=w2693) -> (x .and. y?=w2696:bool)
                    }
                  }
                  frame #7 {
                    n1888 = property on="Trap D (MHz)" class="DigNum (strict)"("Val(Sgnl)"=w2699) -> ()  [unwired: 2 in, 2 out]
                  }
                }
              }
            }
          }
          frame #8 {
            n1889 = local read "Save ave N"() -> (w2701:dbl)
            n1890 = case shown="False" "W/ Offset 2" {
              tunnel: w2702 -> [_ w2709]
              tunnel: w2701 -> [_ w2708]
              tunnel: w2700 -> [w2704 _]
              frame False {
                n1891 = case shown="False" w2704 {
                  frame False {
                    n1892 = Multiply(x="Cal read wait (s)", y=u32 1000 ("milliseconds to wait")) -> (x*y=w2706:u32)
                    n1893 = Wait (ms)(milliseconds to wait=w2706) -> ()  [unwired: 1 out]
                  }
                  frame True {
                  }
                }
              }
              frame True {
                n1894 = stacked-sequence {
                  tunnel: w2709 -> [_ _ _ _ _ _ _ _ _ w2730 _ _]
                  tunnel: w2708 -> [_ _ _ _ _ _ _ _ _ w2728 _ _]
                  frame #0 {
                    n1895 = property on="Save ave N" class="DigNum (strict)"("Val(Sgnl)"=1.0 ("Value (Signaling)")) -> ()  [unwired: 2 in, 2 out]
                  }
                  frame #1 {
                    n1896 = Wait (ms)(milliseconds to wait=u32 500) -> ()  [unwired: 1 out]
                  }
                  frame #2 {
                    n1897 = property on="Trap D (MHz)" class="DigNum (strict)"("Val(Sgnl)"="Offset 2 Start (MHz)") -> ()  [unwired: 2 in, 2 out]
                    n1898 = Replace Array Subset(array=u32[] [0] ("Index Values"), new element="Offset 2 Set", index=0) -> (w2714:u32[])
                    n1899 = property on="Saved AOD Raster Scan Parameter Sets" class="Arr (strict)"("Index Values"=w2714) -> ()  [unwired: 2 in, 2 out]
                  }
                  frame #3 {
                    n1900 = Wait (ms)(milliseconds to wait=u32 500) -> ()  [unwired: 1 out]
                  }
                  frame #4 {
                    n1901 = property on="Load parameters" class="Bool (strict)"("Val(Sgnl)"=TRUE ("Value (Signaling)")) -> ()  [unwired: 2 in, 2 out]
                  }
                  frame #5 {
                    n1902 = Wait (ms)(milliseconds to wait=u32 500) -> ()  [unwired: 1 out]
                  }
                  frame #6 {
                    n1903 = property on="Trap Raster Scan" class="Bool (strict)"("Val(Sgnl)"=TRUE ("Value (Signaling)")) -> ()  [unwired: 2 in, 2 out]
                  }
                  frame #7 {
                    n1904 = Wait (ms)(milliseconds to wait=u32 2000) -> ()  [unwired: 1 out]
                  }
                  frame #8 {
                    n1905 = while {
                      stop <- w2723 stop-if-true
                      n1906 = local read "Raster Scanning..."() -> (w2726:bool)
                      n1907 = local read "Saving..."() -> (w2724:bool)
                      n1908 = Wait (ms)(milliseconds to wait=u32 100) -> ()  [unwired: 1 out]
                      n1909 = Not(x=w2724) -> (.not. x?=w2722:bool)
                      n1910 = Not(x=w2726) -> (.not. x?=w2725:bool)
                      n1911 = And(x=w2725, y=w2722) -> (x .and. y?=w2723:bool)
                    }
                  }
                  frame #9 {
                    n1912 = property on="Trap D (MHz)" class="DigNum (strict)"("Val(Sgnl)"=w2730) -> ()  [unwired: 2 in, 2 out]
                    n1913 = property on="Saved AOD Raster Scan Parameter Sets" class="Arr (strict)"("Index Values"=u32[] [0]) -> ()  [unwired: 2 in, 2 out]
                    n1914 = property on="Save ave N" class="DigNum (strict)"("Val(Sgnl)"=w2728) -> ()  [unwired: 2 in, 2 out]
                  }
                  frame #10 {
                    n1915 = Wait (ms)(milliseconds to wait=u32 500) -> ()  [unwired: 1 out]
                  }
                  frame #11 {
                    n1916 = property on="Load parameters" class="Bool (strict)"("Val(Sgnl)"=TRUE ("Value (Signaling)")) -> ()  [unwired: 2 in, 2 out]
                  }
                }
              }
            }
          }
          frame #9 {
            n1917 = property on="Read Cal" class="Bool (strict)"("Val(Sgnl)"=TRUE ("Value (Signaling)")) -> ()  [unwired: 2 in, 2 out]
          }
          frame #10 {
            n1918 = Wait (ms)(milliseconds to wait=u32 1000) -> ()  [unwired: 1 out]
          }
          frame #11 {
            n1919 = property on="Fish" class="Bool (strict)"("Val(Sgnl)"=TRUE ("Value (Signaling)")) -> ()  [unwired: 2 in, 2 out]
          }
        }
        n1920 = local write "Cal/Data Acq. Spot"(FALSE ("Cal/Data Acq. Spot")) -> ()
      }
      event "Dump Beads": Value Change {
        n1921 = event-data() -> ()  [unwired: 1 in, 5 out]
        n1922 = flat-sequence {
          tunnel: ["Dump spot flow on?"] -> w2736
          tunnel: [w2748] -> w2737
          tunnel: w2736 -> [w2748]
          tunnel: w2740 -> [w2753]
          tunnel: w2739 -> [w2752]
          tunnel: [w2750] -> w2738
          tunnel: w2737 -> [w2750]
          tunnel: w2738 -> [w2764]
          frame #0 {
            w2741 = FALSE ("Value (Signaling)")
            n1923 = local read "Saving..."() -> (w2743:bool)
            n1924 = local write "Dump Beads"(FALSE ("Dump Beads")) -> ()
            n1925 = property on="Inject Pump 3" class="Bool (strict)"("Val(Sgnl)"=w2741) -> ()  [unwired: 2 in, 2 out]
            n1926 = property on="Inject Pump 1" class="Bool (strict)"("Val(Sgnl)"=w2741) -> ()  [unwired: 2 in, 2 out]
            n1927 = local write "Stop Saving"(w2743) -> ()
            n1928 = local write "Fish"(w2741) -> ()
          }
          frame #1 {
            w2744 = TRUE
            w2745 = FALSE ("Fl. Triggered...")
            n1929 = case shown="True" "Dump spot flow on?" {
              frame False {
              }
              frame True {
                n1930 = property on="Sample Channel\nFlow" class="Bool (strict)"("Val(Sgnl)"=TRUE ("Stage Moving")) -> ()  [unwired: 2 in, 2 out]
              }
            }
            n1931 = local write "Fl. Triggered..."(w2745) -> ()
            n1932 = local write "Tether"(w2745) -> ()
            n1933 = local write "Multiple tether"(w2745) -> ()
            n1934 = local write "Good tether"(w2745) -> ()
            n1935 = property on="Green ON/Interlacing" class="Bool (strict)"("Val(Sgnl)"=w2745) -> ()  [unwired: 2 in, 2 out]
            n1936 = property on="Trap Pos. FB ON" class="Bool (strict)"("Val(Sgnl)"=w2745) -> ()  [unwired: 2 in, 2 out]
            n1937 = property on="Trap Trig. Fl." class="Bool (strict)"("Val(Sgnl)"=w2745) -> ()  [unwired: 2 in, 2 out]
            n1938 = local write "Bad fit"(w2745) -> ()
            n1939 = local write "Hysteresis"(w2745) -> ()
            n1940 = property on="Fl. Triggered..." class="Bool (strict)"("Val(Sgnl)"=w2745) -> ()  [unwired: 2 in, 2 out]
            n1941 = local write "Restart DMA? (AOD)"(w2744) -> ()
            n1942 = local write "Save scans"(w2744) -> ()
            n1943 = property on="Dip for Protein" class="Bool (strict)"("Val(Sgnl)"=w2745) -> ()  [unwired: 2 in, 2 out]
            n1944 = property on="Pause dwell" class="Bool (strict)"("Val(Sgnl)"=w2745) -> ()  [unwired: 2 in, 2 out]
          }
          frame #2 {
            n1945 = property on="Trap Pos. FB Offset Factor" class="DigNum (strict)"("Val(Sgnl)"=i64 0 ("Value (Signaling)")) -> ()  [unwired: 2 in, 2 out]
          }
          frame #3 {
            n1946 = local read "Saved Stage Positions"() -> (w2754:dbl[][])
            n1947 = Array Subset(array=w2754, index (row)=3 ("index"), length (row)=1 ("length"), index (col)=1 ("index"), length (col)=3 ("length")) -> (w2759:dbl[][])
            n1948 = local write "Stage Moving"(TRUE ("Stage Moving")) -> ()
            n1949 = Reshape Array(w2759, 3 ("dimension size")) -> (w2757:dbl[])
            n1950 = Array To Cluster(array=w2757) -> (cluster=w2756:cluster{"[0]":dbl, "[1]":dbl, "[2]":dbl})
            n1951 = call "Set Stage Position.vi"("Position"=w2756, "error in"=w2752, "VISA resource name in"=w2753) -> ()  [unwired: 3 out]
          }
          frame #4 {
            w2765 = FALSE ("Value (Signaling)")
            n1952 = case shown="True" w2764 {
              frame False {
              }
              frame True {
                n1953 = property on="Sample Channel\nFlow" class="Bool (strict)"("Val(Sgnl)"=FALSE ("Stage Moving")) -> ()  [unwired: 2 in, 2 out]
              }
            }
            n1954 = property on="Trap 1 (ON/OFF)" class="Bool (strict)"("Val(Sgnl)"=w2765) -> ()  [unwired: 2 in, 2 out]
            n1955 = property on="Trap 2 (ON/OFF)" class="Bool (strict)"("Val(Sgnl)"=w2765) -> ()  [unwired: 2 in, 2 out]
            n1956 = call <vilib>:"Beep.vi"() -> ()  [unwired: 3 in, 9 out]
            n1957 = local write "Fish"(FALSE ("Fish for Tether")) -> ()
          }
          frame #5 {
            n1958 = property on="Move Cap. 2 (ADig Top)" class="Bool (strict)"("Val(Sgnl)"=TRUE ("Value (Signaling)")) -> ()  [unwired: 2 in, 2 out]
            n1959 = property on="Tab Control" class="TabCtl (strict)"("Val(Sgnl)"=T34."Status" ("Value (Signaling)")) -> ()  [unwired: 2 in, 2 out]
          }
        }
      }
      event "Dip for Protein": Value Change {
        n1960 = event-data() -> ()  [unwired: 1 in, 5 out]
        n1961 = case shown="True" "Dip for Protein" {
          tunnel: w2771 -> [_ w2773]
          tunnel: w2770 -> [_ w2772]
          frame False {
          }
          frame True {
            n1962 = while {
              tunnel: w2773 -> [w2784]
              tunnel: w2772 -> [w2783]
              i -> [w2779]
              stop <- w2774 stop-if-true
              n1963 = Increment(x=w2779) -> (x+1=→"Dip #":i32)
              n1964 = flat-sequence {
                tunnel: w2783 -> [w2795]
                tunnel: w2784 -> [w2796]
                tunnel: [w2796] -> w2788
                tunnel: [w2795] -> w2787
                tunnel: [w2789] -> w2775
                tunnel: [w2801] -> w2782
                tunnel: [w2802] -> w2781
                tunnel: w2788 -> [w2803]
                tunnel: w2787 -> [w2804]
                tunnel: [w2799] -> w2776
                tunnel: w2775 -> [w2799]
                tunnel: [w2812] -> w2786
                tunnel: w2782 -> [w2812]
                tunnel: [w2811] -> w2785
                tunnel: w2781 -> [w2811]
                tunnel: [w2808] -> w2780
                tunnel: [w2807] -> w2777
